vi "zcom ff and fb.vi"(10 "projections":T2) -> (2 "Cluster":T1)   [LabVIEW 2010]
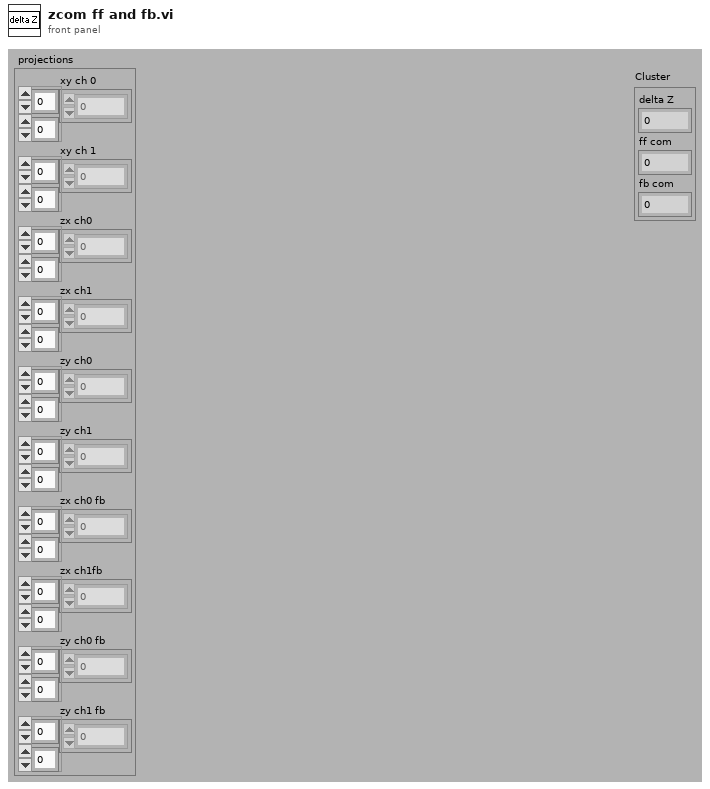
[diagram p1: front panel]
types:
  T1 = cluster{"delta Z":dbl, "ff com":dbl, "fb com":dbl}
  T2 = cluster{"xy ch 0":u16[][], "xy ch 1":u16[][], "zx ch0":u16[][], "zx ch1":u16[][], "zy ch0":u16[][], "zy ch1":u16[][], "zx ch0 fb":u16[][], "zx ch1fb":u16[][], "zy ch0 fb":u16[][], "zy ch1 fb":u16[][]}
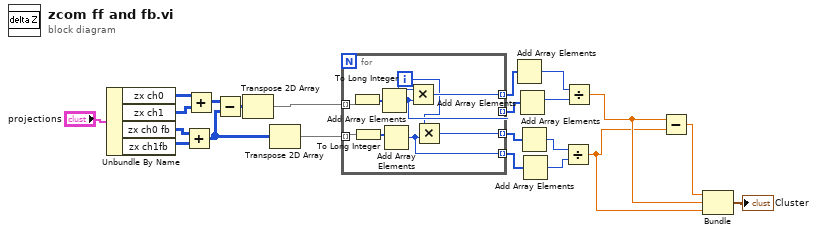
[diagram p0: block diagram]
diagram:
  n1 = Unbundle By Name("projections") -> ("zx ch0"=w21:u16[][], "zx ch1"=w20:u16[][], "zx ch0 fb"=w19:u16[][], "zx ch1fb"=w18:u16[][])
  n2 = Add(x=w19, y=w18) -> (x+y=w16:u16[][])
  n3 = Add(x=w21, y=w20) -> (x+y=w17:u16[][])
  n4 = Subtract(x=w17, y=w16) -> (x-y=w15:u16[][])
  n5 = Transpose 2D Array(2D array=w15) -> (transposed array=w6:u16[][])
  n6 = Transpose 2D Array(2D array=w16) -> (transposed array=w5:u16[][])
  n7 = for {
    tunnel: w5 -> [w29] mode=indexing
    tunnel: w6 -> [w31] mode=indexing
    tunnel: [w27] -> w14 mode=indexing
    tunnel: [w26] -> w13 mode=indexing
    tunnel: [w24] -> w12 mode=indexing
    tunnel: [w23] -> w11 mode=indexing
    i -> [w25]
    n8 = To Long Integer(number=w31) -> (32bit integer=w30:i32[])
    n9 = To Long Integer(number=w29) -> (32bit integer=w28:i32[])
    n10 = Add Array Elements(numeric array=w30) -> (sum=w26:i32)
    n11 = Add Array Elements(numeric array=w28) -> (sum=w23:i32)
    n12 = Multiply(x=w25, y=w26) -> (x*y=w27:i32)
    n13 = Multiply(x=w25, y=w23) -> (x*y=w24:i32)
  }
  n14 = Add Array Elements(numeric array=w14) -> (sum=w10:i32)
  n15 = Add Array Elements(numeric array=w13) -> (sum=w9:i32)
  n16 = Add Array Elements(numeric array=w12) -> (sum=w8:i32)
  n17 = Add Array Elements(numeric array=w11) -> (sum=w7:i32)
  n18 = Divide(x=w8, y=w7) -> (x/y=w2:dbl)
  n19 = Divide(x=w10, y=w9) -> (x/y=w3:dbl)
  n20 = Subtract(x=w3, y=w2) -> (x-y=w4:dbl)
  n21 = Bundle(w4, w3, w2) -> (→"Cluster":cluster{dbl, dbl, dbl})  [unwired: 1 in]
